vi "PreparePassReceiverRole.vi"(5 "Striker/2ndStriker":T1, 6 "Tactic index in":i32, 7 "first call":bool, 8 "error in (no error)":errorcluster, 10 "Game in":refnum<class "Game.lvclass">, 11 "PreparePassReceiverRole in":refnum<class "PreparePassReceiverRole.lvclass">) -> (0 "error out":errorcluster, 1 "Robot out":refnum<class "Robot.lvclass">, 2 "Game out":refnum<class "Game.lvclass">, 3 "PreparePassReceiverRole out":refnum<class "PreparePassReceiverRole.lvclass">, 4 "tactic index":i32)   [LabVIEW 2020, in "PreparePassReceiverRole.lvclass"]
uses:
  PreparePassReceiverRole.lvclass
  C:/Users/anton/Desktop/RoboIME/IC/SSL_AI/Role_class/Role.lvclass
  Game_class/Game.lvclass
  Robot_class/Robot.lvclass
  PreparePassReceiverEnum.ctl
  Role_class/Role.lvclass/Role.ctl
  PositionToReceivePassTactic_class/PositionToReceivePassTactic.lvclass/PositionToReceivePassTactic.ctl
  PositionToReceivePassTactic_class/Read States.vi
  Role_class/Read RobotRef.vi
  Role_class/Read Tacticbook.vi
  Role_class/Write Tacticbook.vi
  Role_class/Write tactic_index.vi
  Tacticbook_class/Tacticbook.lvclass
  PositionToReceivePassTactic_class/PositionToReceivePassTactic.lvclass
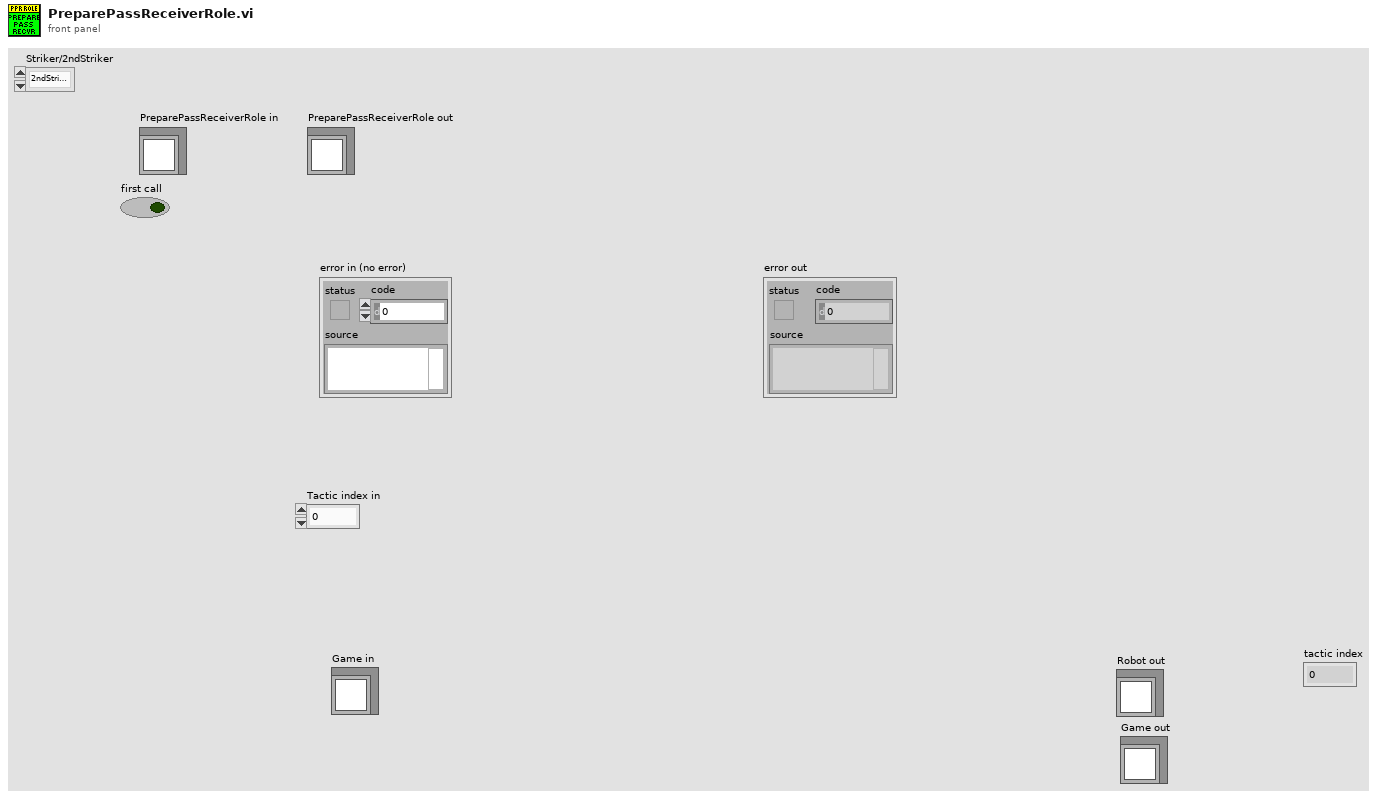
[diagram p1: front panel]
types:
  T1 = typedef "PreparePassReceiverEnum.ctl" = enum16{"2ndStrikerDPass", "2ndStriker", "Striker"}
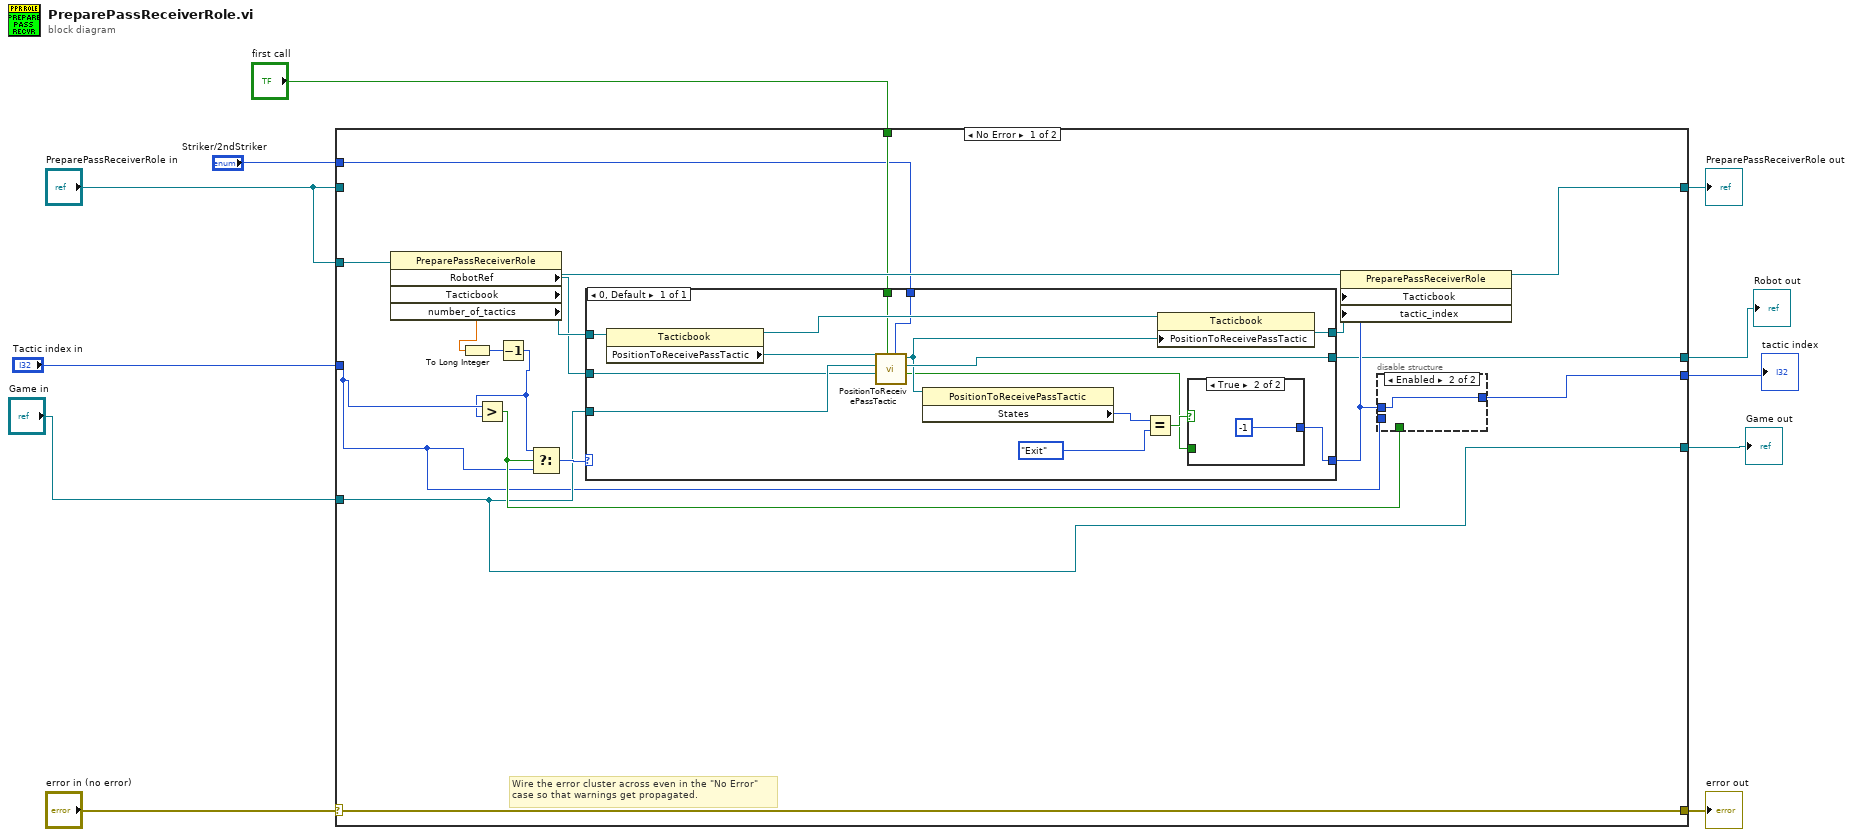
[diagram p0: block diagram]
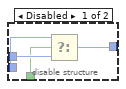
[diagram p2: hidden frame]
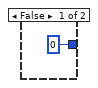
[diagram p3: hidden frame]
diagram:
  n1 = case shown="No Error" "error in (no error)" {
    selector: "error in (no error)" -> [w30 w54]
    tunnel: [w30 w54] -> w10
    tunnel: [w18 w53] -> w9
    tunnel: "PreparePassReceiverRole in" -> [_ w53]
    tunnel: "first call" -> [w23 _]
    tunnel: [w22 _] -> w7
    tunnel: [w21 _] -> w6
    tunnel: "Game in" -> [w20 _]
    tunnel: [w20 _] -> w4
    tunnel: "PreparePassReceiverRole in" -> [w19 _]
    tunnel: "Tactic index in" -> [w17 _]
    tunnel: "Striker/2ndStriker" -> [w16 _]
    frame No Error {
      # "Wire the error cluster across even in the \"No Error\"\ncase so that warnings get propagated."
      n2 = property class="PreparePassReceiverRole"(reference=w19) -> (reference out=w29:refnum<class "PreparePassReceiverRole.lvclass">, "RobotRef"=w12:refnum<class "Robot.lvclass">, "Tacticbook"=w28:refnum<class "Tacticbook.lvclass">, "number_of_tactics"=w15:dbl)  [unwired: 1 in, 1 out]
      n3 = To Long Integer(number=w15) -> (32bit integer=w14:i32)
      n4 = Decrement(x=w14) -> (x-1=w13:i32)
      n5 = Greater?(x=w17, y=w13) -> (0:w24:bool)
      n6 = Select(t=w13, s=w24, f=w17) -> (s? t:f=w25:i32)
      n7 = case shown="0, Default" w25 {
        tunnel: [w42] -> w26
        tunnel: w28 -> [w50]
        tunnel: [w49] -> w22
        tunnel: [w47] -> w27
        tunnel: w20 -> [w45]
        tunnel: w23 -> [w41]
        tunnel: w16 -> [w38]
        tunnel: w12 -> [w36]
        frame 0, Default {
          n8 = property class="Tacticbook"(reference=w50) -> (reference out=w48:refnum<class "Tacticbook.lvclass">, "PositionToReceivePassTactic"=w46:refnum<class "PositionToReceivePassTactic.lvclass">)  [unwired: 1 in, 1 out]
          n9 = call "PositionToReceivePassTactic.vi"("Striker/2ndStriker"=w38, "first call"=w41, "Robot"=w36, "Game in"=w45, "PositionToReceivePassTactic in"=w46) -> ("Sucsses"=w37:bool, "Robot out"=w49:refnum<class "Robot.lvclass">, "PositionToReceivePassTactic out"=w44:refnum<class "PositionToReceivePassTactic.lvclass">)  [unwired: 3 in, 1 out]
          n10 = property class="PositionToReceivePassTactic"(reference=w44) -> ("States"=w39:enum16{"ReceivePass", "Exit"})  [unwired: 1 in, 2 out]
          n11 = Equal?(x=w39, y=enum16{"ReceivePass", "Exit"}."Exit" ("States")) -> (x = y?=w43:bool)
          n12 = property class="Tacticbook"(reference=w48, "PositionToReceivePassTactic"=w44) -> (reference out=w47:refnum<class "Tacticbook.lvclass">)  [unwired: 1 in, 1 out]
          n13 = case shown="True" w43 {
            tunnel: [0 -1] -> w42
            tunnel: w37 -> [_ _]
            frame False {
            }
            frame True {
            }
          }
        }
      }
      n14 = property class="PreparePassReceiverRole"(reference=w29, "Tacticbook"=w27, "tactic_index"=w26) -> (reference out=w18:refnum<class "PreparePassReceiverRole.lvclass">)  [unwired: 1 in, 1 out]
      n15 = disable-structure shown="Enabled" {
        disable-tunnel: w26 -> [w34 w35]
        disable-tunnel: w24 -> [w33 _]
        disable-tunnel: [w32 w35] -> w21
        disable-tunnel: w17 -> [w31 _]
        frame Disabled {
          n16 = Select(t=w31, s=w33, f=w34) -> (s? t:f=w32:i32)
        }
        frame Enabled {
        }
      }
    }
    frame Error {
    }
  }
  "error out" <- w10
  "PreparePassReceiverRole out" <- w9
  "Robot out" <- w7
  "Game out" <- w4
  "tactic index" <- w6
